vi "Receive All Signals.vi"(8 "error in":errorcluster, 11 "PCAN in":refnum<class "PCAN.lvclass">) -> (0 "error out":errorcluster, 2 "All Signals":T1, 3 "PCAN out":refnum<class "PCAN.lvclass">)   [LabVIEW 2023, in "PCAN.lvclass"]
uses:
  PCAN.lvclass
  PCAN.lvclass/PCAN.ctl
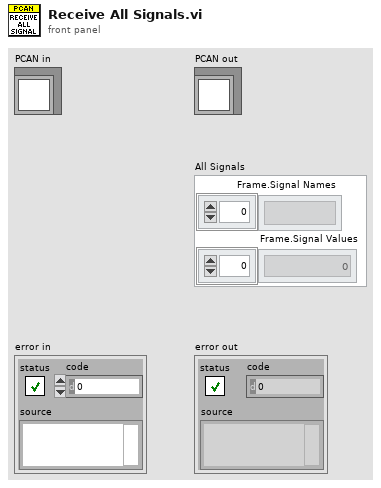
[diagram p1: front panel]
types:
  T1 = cluster{"Frame.Signal Names":string[], "Frame.Signal Values":dbl[]}
  T2 = cluster{"Signal Names":string[], "Signal Values":dbl[]}
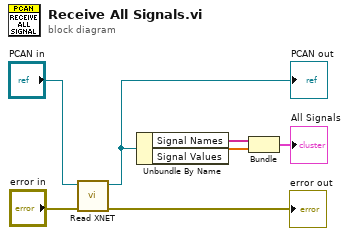
[diagram p0: block diagram]
diagram:
  n1 = call "Read XNET.vi"("error in"="error in", "PCAN in"="PCAN in") -> ("error out"=→"error out":errorcluster, "PCAN out"=w4:refnum<class "PCAN.lvclass">)  [unwired: 8 in]
  "PCAN out" <- w4
  n2 = Unbundle By Name(w4) -> ("Signal Names"=w3:string[], "Signal Values"=w2:dbl[])
  n3 = Bundle("Signal Names"=w3, "Signal Values"=w2) -> (→"All Signals":T2)  [unwired: 1 in]
